vi "Report.vi"(8 "error in (no error)":errorcluster) -> (0 "error out":errorcluster)   [LabVIEW 2020]
uses:
  Global_Variable/A131258.vi
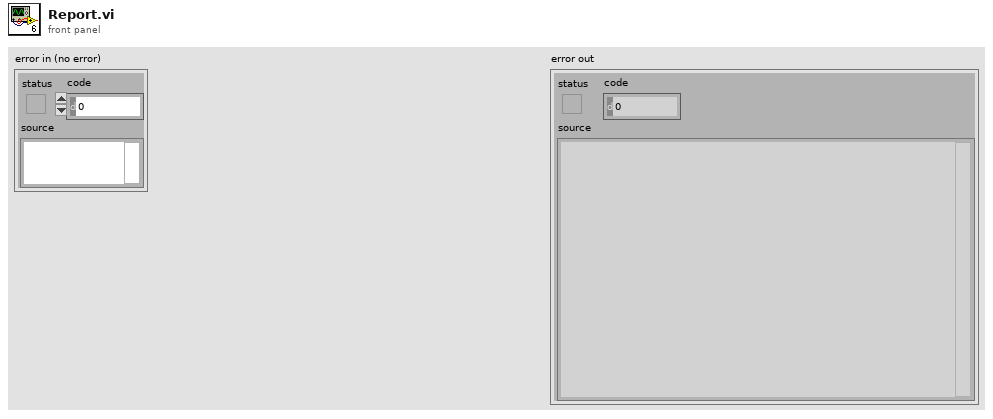
[diagram p1: front panel]
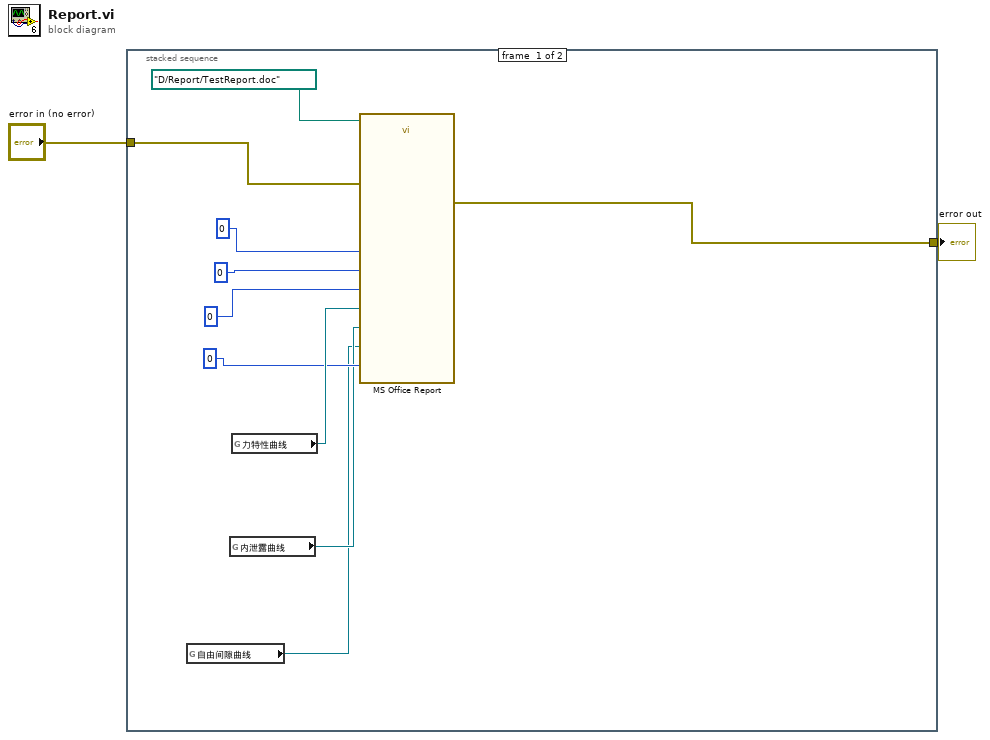
[diagram p0: block diagram]
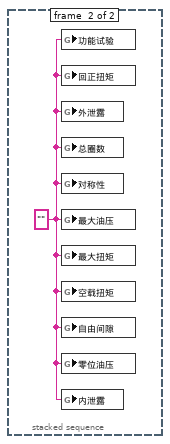
[diagram p2: hidden frame]
diagram:
  n1 = stacked-sequence {
    tunnel: [w11 _] -> w2
    tunnel: "error in (no error)" -> [w10 _]
    frame #0 {
      n2 = global read "A131258.vi" "自由间隙曲线"() -> (w3:refnum<vi>)
      n3 = global read "A131258.vi" "内泄露曲线"() -> (w4:refnum<vi>)
      n4 = global read "A131258.vi" "力特性曲线"() -> (w9:refnum<vi>)
      n5 = call "MS Office Report"("Path to Save Report"=path "D:/Report/TestReport.doc", "产品型号"=0, "产品编号"=0, "操作员"=0, "曲线"=w9, "曲线2"=w4, "error in (no error)"=w10, "曲线3"=w3, "检验员"=0) -> ("error out"=w11:errorcluster)  [unwired: 17 in, 1 out]
    }
    frame #1 {
      w13 = "" ("内泄露")
      n6 = global write "检测结果.vi" "功能试验"(w13) -> ()
      n7 = global write "检测结果.vi" "回正扭矩"(w13) -> ()
      n8 = global write "检测结果.vi" "外泄露"(w13) -> ()
      n9 = global write "检测结果.vi" "总圈数"(w13) -> ()
      n10 = global write "检测结果.vi" "对称性"(w13) -> ()
      n11 = global write "检测结果.vi" "最大油压"(w13) -> ()
      n12 = global write "检测结果.vi" "最大扭矩"(w13) -> ()
      n13 = global write "检测结果.vi" "空载扭矩"(w13) -> ()
      n14 = global write "检测结果.vi" "自由间隙"(w13) -> ()
      n15 = global write "检测结果.vi" "零位油压"(w13) -> ()
      n16 = global write "检测结果.vi" "内泄露"(w13) -> ()
    }
  }
  "error out" <- w2
